vi "PWM_TS.vi"(8 "error out 2":errorcluster) -> (0 "error out 3":errorcluster, 2 "Result (bool)":bool, 3 "Message OUT":string, 10 "Analysis Leg":i32, 11 "Active Leg":i32)   [LabVIEW 2022 SP3]
uses:
  HMP4000 Communication/HMP4040_ChannelControl.ctl
  <vilib>/DAQmx/read.llb/DAQmx Read (Analog 1D Wfm NChan NSamp).vi
  <vilib>/DAQmx/miscellaneous.llb/DAQmx Fill In Error Info.vi
panel:
  in  "Message IN":string=" "
  out "Result (color)":u32(colorbox)
  out "Waveforms":T1
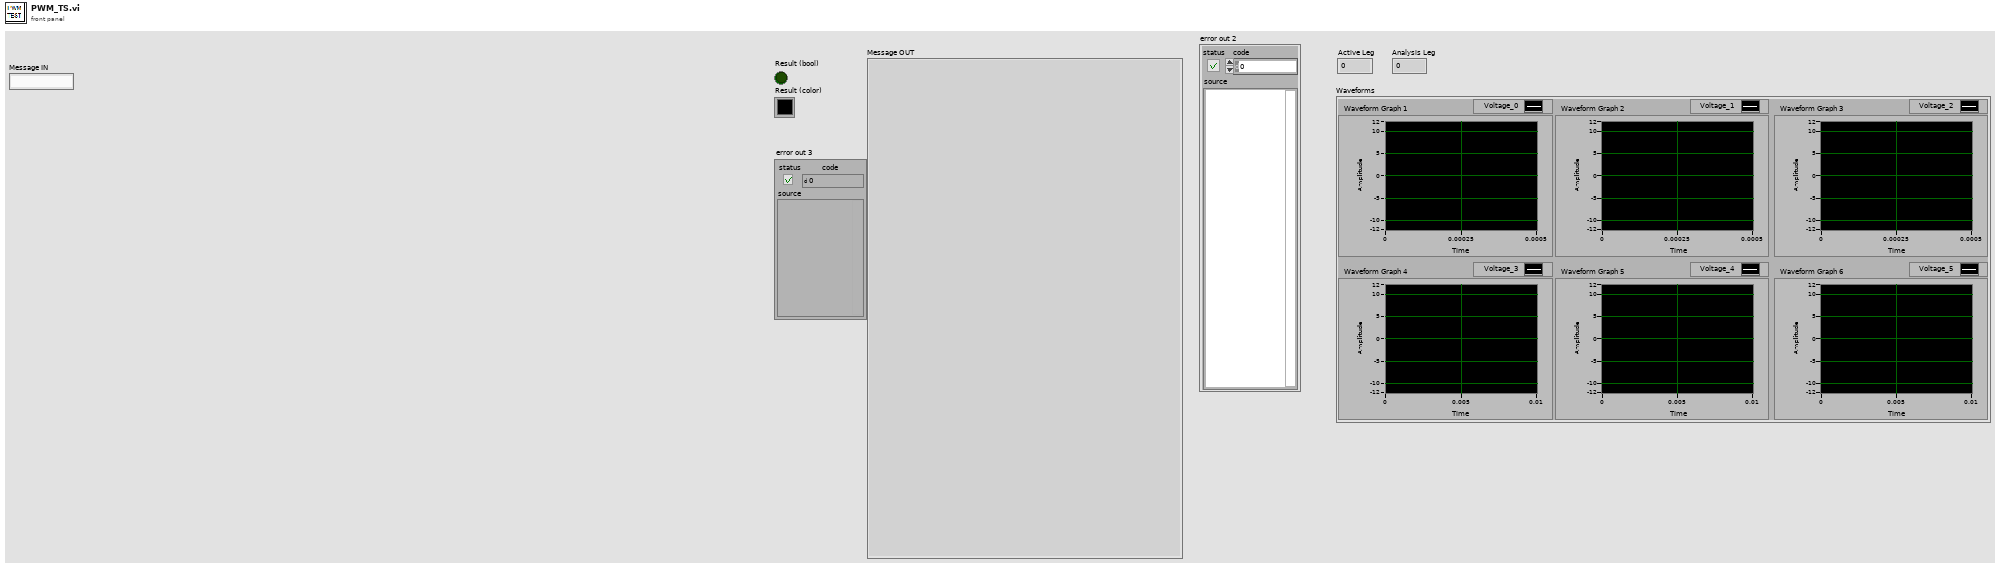
[diagram p1: front panel]
types:
  T1 = cluster{"Waveform Graph 1":waveform(dbl), "Waveform Graph 2":waveform(dbl), "Waveform Graph 3":waveform(dbl), "Waveform Graph 4":waveform(dbl), "Waveform Graph 5":waveform(dbl), "Waveform Graph 6":waveform(dbl)}
  T2 = typedef "HMP4040_ChannelControl.ctl" = cluster{"CH1 Voltage":dbl, "CH1 Current":dbl, "CH1 Output":bool, "CH2 Voltage":dbl, "CH2 Current":dbl, "CH2 Output":bool, "CH3 Voltage":dbl, "CH3 Current":dbl, "CH3 Output":bool, "CH4 Voltage":dbl, "CH4 Current":dbl, "CH4 Output":bool, "Master Output":bool}
  T3 = cluster{"data[0]":waveform(dbl), "data[1]":waveform(dbl), "data[2]":waveform(dbl), "data[3]":waveform(dbl), "data[4]":waveform(dbl), "data[5]":waveform(dbl)}
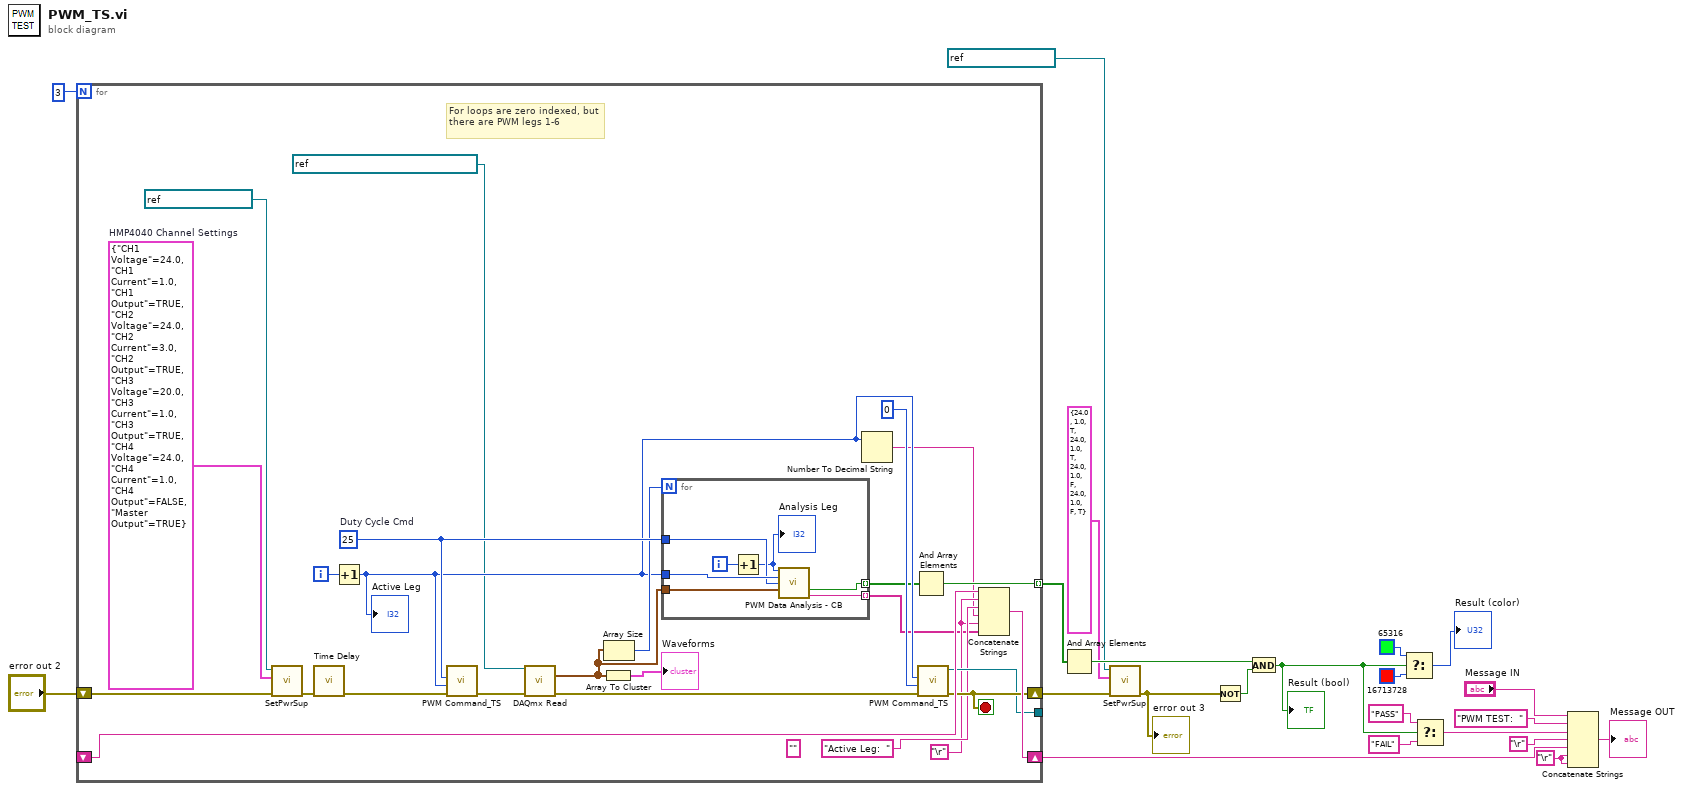
[diagram p0: block diagram]
diagram:
  w12 = "\r"
  n1 = for {
    N: 3 -> [_]
    tunnel: [w47] -> w5 mode=indexing
    shift-right: [w46] -> w6
    shift-left: _ -> [w45]
    tunnel: [w36] -> _
    shift-right: [w40] -> w4
    shift-left: "error out 2" -> [w29]
    i -> [w42]
    stop <- w40 stop-if-true
    (unwired) ""
    w28 = T2 {"CH1 Voltage"=24.0, "CH1 Current"=1.0, "CH1 Output"=TRUE, "CH2 Voltage"=24.0, "CH2 Current"=3.0, "CH2 Output"=TRUE, "CH3 Voltage"=20.0, "CH3 Current"=1.0, "CH3 Output"=TRUE, "CH4 Voltage"=24.0, "CH4 Current"=1.0, "CH4 Output"=FALSE, "Master Output"=TRUE}  # HMP4040 Channel Settings
    w32 = "\r"
    w43 = 25  # Duty Cycle Cmd
    # "For loops are zero indexed, but there are PWM legs 1-6"
    n2 = call "SetPwrSup.vi"("error in (no error)"=w29, "HMP4040 Channel Settings"=w28, "HMP4040 IN"=refnum<visa-resource-name> "HMP4040_FTS2" ("HMP4040_IN")) -> ("error out"=w27:errorcluster)  [unwired: 7 in, 1 out]
    n3 = call "Time Delay"("error in (no error)"=w27) -> ("error out"=w26:errorcluster)  [unwired: 10 in]
    n4 = Increment(x=w42) -> (x+1=w33:i32)
    "Active Leg" <- w33
    n5 = call "PWM Command_TS.vi"("error in (no error) 2"=w26, "Leg"=w33, "Duty Cycle"=w43) -> ("error out"=w35:errorcluster)  [unwired: 1 in, 7 out]
    n6 = call-poly <vilib>:"DAQmx Read.vi"("task/channels in"=refnum<k21> "FTS2_PWMInput_CarrierBoard", "error in"=w35) -> ("data"=w37:waveform(dbl)[], "error out"=w41:errorcluster)  [unwired: 11 in, 1 out]
    n7 = Array To Cluster(array=w37) -> (cluster=→"Waveforms":T3)
    n8 = Array Size(array=w37) -> (size(s)=w38:i32)
    n9 = for {
      N: w38 -> [_]
      tunnel: w43 -> [w51]
      tunnel: w37 -> [w52]
      tunnel: w33 -> [w54]
      tunnel: [w50] -> w25 mode=indexing
      tunnel: [w49] -> w24 mode=indexing
      i -> [w53]
      n10 = Increment(x=w53) -> (x+1=w48:i32)
      "Analysis Leg" <- w48
      n11 = call "PWM Data Analysis - CB.vi"("Analysis Leg"=w48, "Active Leg"=w54, "Duty Cycle"=w51, "Waveform"=w52) -> ("Result (Boolean)"=w49:bool, "Message"=w50:string)  [unwired: 10 in]
    }
    n12 = Number To Decimal String(number=w33) -> (decimal integer string=w31:string)  [unwired: 1 in]
    n13 = And Array Elements(Boolean array=w24) -> (logical AND=w47:bool)
    n14 = call "PWM Command_TS.vi"("error in (no error) 2"=w41, "Leg"=0 ("Duty Cycle"), "Duty Cycle"=w33) -> ("error out"=w40:errorcluster, "VISA Refnum out"=w36:refnum<visa-resource-name>)  [unwired: 1 in, 6 out]
    n15 = Concatenate Strings(w45, w32, "Active Leg:  ", w31, w32, w25) -> (w46:string)
  }
  n16 = And Array Elements(Boolean array=w5) -> (logical AND=w13:bool)
  n17 = call "SetPwrSup.vi"("error in (no error)"=w4, "HMP4040 Channel Settings"=T2 {"CH1 Voltage"=24.0, "CH1 Current"=1.0, "CH1 Output"=TRUE, "CH2 Voltage"=24.0, "CH2 Current"=1.0, "CH2 Output"=TRUE, "CH3 Voltage"=24.0, "CH3 Current"=1.0, "CH3 Output"=FALSE, "CH4 Voltage"=24.0, "CH4 Current"=1.0, "CH4 Output"=FALSE, "Master Output"=TRUE}, "HMP4040 IN"=refnum<visa-resource-name> "HMP4040_FTS2" ("HMP4040_IN")) -> ("error out"=w3:errorcluster)  [unwired: 7 in, 1 out]
  "error out 3" <- w3
  n18 = Not(x=w3) -> (.not. x?=w15:bool)
  n19 = And(x=w13, y=w15) -> (x .and. y?=w14:bool)
  "Result (bool)" <- w14
  n20 = Select(t=u32 65316 ("Result (color)"), s=w14, f=u32 16713728 ("Result (color)")) -> (s? t:f=→"Result (color)":u32)
  n21 = Select(t="PASS", s=w14, f="FAIL") -> (s? t:f=w7:string)
  n22 = Concatenate Strings("Message IN", "PWM TEST:  ", w7, "\r", w6, w12, w12) -> (→"Message OUT":string)
